vi "Read DeviceSignals.vi"(8 "error in (no error)":errorcluster, 11 "Configuration in":refnum<class "Configuration.lvclass">) -> (0 "error out":errorcluster, 2 "DeviceSingals":string[][](array[string]), 3 "Configuration out":refnum<class "Configuration.lvclass">)   [LabVIEW 2023, in "Configuration.lvlib" / "Configuration.lvclass"]
doc: "SLL->Read DeviceSignals -> This routine accesses the device specific data Row 0 represents the headers, and the remaining rows are the specific signals, this routine should be called in <b>Parse Signal List</b>"
uses:
  Library/Configuration.lvclass
  Library/Configuration.lvclass/Configuration.ctl
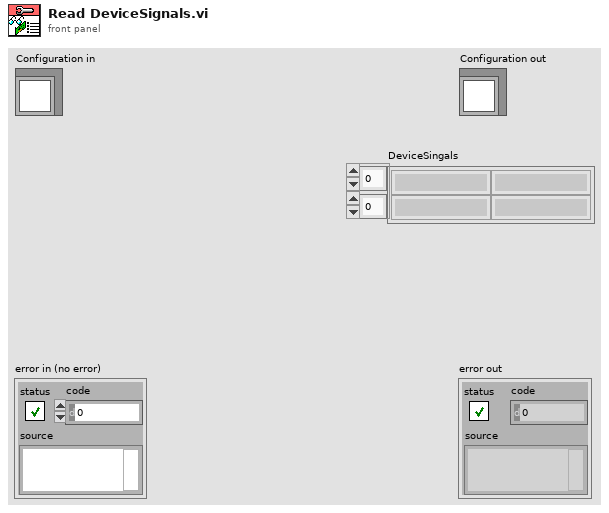
[diagram p1: front panel]
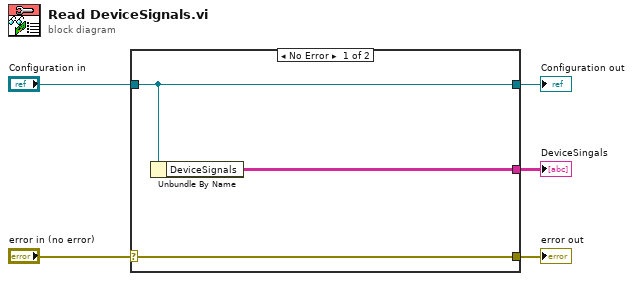
[diagram p0: block diagram]
diagram:
  n1 = case shown="No Error" "error in (no error)" {
    selector: "error in (no error)" -> [w8 w9]
    tunnel: [w8 w9] -> w4
    tunnel: [w7 w10] -> w2
    tunnel: "Configuration in" -> [w7 w10]
    tunnel: [w6 _] -> w1
    frame No Error {
      n2 = Unbundle By Name(w7) -> ("DeviceSignals"=w6:string[][])
    }
    frame Error {
    }
  }
  "error out" <- w4
  "Configuration out" <- w2
  "DeviceSingals" <- w1
